vi "DelayPeriod.vi"(8 "error in (no error)":errorcluster, 11 "TrialBasedExperiment in":refnum<class "WhiteNoiseOrientationDetection.lvclass">) -> (0 "error out":errorcluster, 2 "Timeout":dbl, 3 "TrialBasedExperiment out":refnum<class "WhiteNoiseOrientationDetection.lvclass">)   [LabVIEW 2014, in "WhiteNoiseOrientationDetection.lvclass"]
uses:
  WhiteNoiseOrientationDetection.lvclass
  WhiteNoiseOrientationDetection.lvclass/WhiteNoiseOrientationDetection.ctl
  Trial Based Experiment Statechart/MatlabExperiment/MatlabExperiment.lvclass
  Matlab API/Matlab API.lvlib
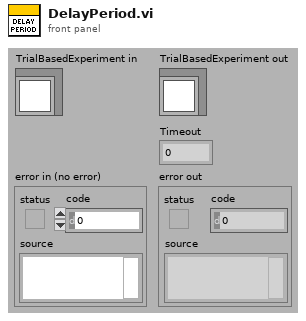
[diagram p1: front panel]
types:
  T1 = cluster{"Intertrial":dbl, "AcquireFixation":dbl, "HoldFixation":dbl, "DelayPeriod":dbl, "ResponsePeriod":dbl}
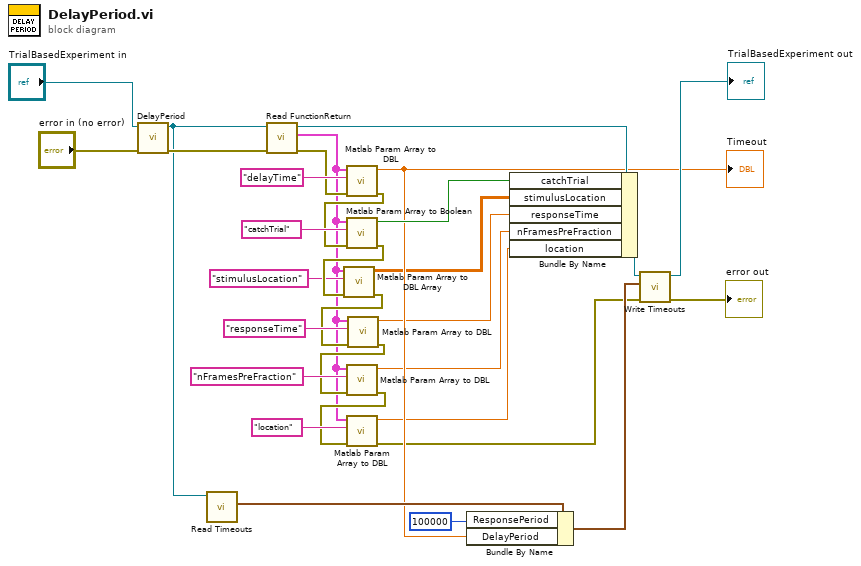
[diagram p0: block diagram]
diagram:
  n1 = call-parent "DelayPeriod.vi"("error in (no error)"="error in (no error)", "TrialBasedExperiment in"="TrialBasedExperiment in") -> ("error out"=w23:errorcluster, "TrialBasedExperiment out"=w22:refnum<class "WhiteNoiseOrientationDetection.lvclass">)  [unwired: 7 in, 1 out]
  n2 = call-dynamic "Read Timeouts.vi"("TrialBasedExperiment in"=w22) -> ("Timeouts"=w21:T1)  [unwired: 8 in, 2 out]
  n3 = call-dynamic "Read FunctionReturn.vi"("error in (no error)"=w23, "MatlabExperiment in"=w22) -> ("error out"=w27:errorcluster, "FunctionReturn"=w1:cluster{"Name":string, "Data":variant}[], "MatlabExperiment out"=w30:refnum<class "WhiteNoiseOrientationDetection.lvclass">)  [unwired: 7 in]
  n4 = call "Matlab Param Array to DBL.vi"("error in (no error)"=w27, "Name"="delayTime", "Matlab Param Array"=w1) -> ("error out"=w26:errorcluster, "data"=w11:dbl)  [unwired: 7 in]
  "Timeout" <- w11
  n5 = call "Matlab Param Array to Boolean.vi"("error in (no error)"=w26, "Name"="catchTrial", "Matlab Param Array"=w1) -> ("error out"=w16:errorcluster, "data"=w29:bool)  [unwired: 7 in]
  n6 = call "Matlab Param Array to DBL Array.vi"("error in (no error)"=w16, "Name"="stimulusLocation", "Matlab Param Array"=w1) -> ("error out"=w12:errorcluster, "data"=w6:dbl[][])  [unwired: 7 in]
  n7 = call "Matlab Param Array to DBL.vi"("error in (no error)"=w12, "Name"="responseTime", "Matlab Param Array"=w1) -> ("error out"=w8:errorcluster, "data"=w10:dbl)  [unwired: 7 in]
  n8 = call "Matlab Param Array to DBL.vi"("error in (no error)"=w8, "Name"="nFramesPreFraction", "Matlab Param Array"=w1) -> ("error out"=w4:errorcluster, "data"=w7:dbl)  [unwired: 7 in]
  n9 = call "Matlab Param Array to DBL.vi"("error in (no error)"=w4, "Name"="location", "Matlab Param Array"=w1) -> ("error out"=w3:errorcluster, "data"=w2:dbl)  [unwired: 7 in]
  n10 = Bundle By Name(cluster=w21, "ResponsePeriod"=100000, "DelayPeriod"=w11) -> (w18:T1)
  n11 = Bundle By Name(cluster=w30, "catchTrial"=w29, "stimulusLocation"=w6, "responseTime"=w10, "nFramesPreFraction"=w7, "location"=w2) -> (w20:refnum<class "WhiteNoiseOrientationDetection.lvclass">)
  n12 = call-dynamic "Write Timeouts.vi"("error in (no error)"=w3, "Timeouts"=w18, "TrialBasedExperiment in"=w20) -> ("error out"=→"error out":errorcluster, "TrialBasedExperiment out"=→"TrialBasedExperiment out":refnum<class "WhiteNoiseOrientationDetection.lvclass">)  [unwired: 7 in]
